vi "CRYView Queue.vi"() -> ()   [LabVIEW 2013]
uses:
  CRYView Global.vi
  SubVI/CRYMain Sub Window Global.vi
panel:
  in  "bVIRefRemove":bool=TRUE
  in  "ResultInCurLibrary":T1={"bResult"=TRUE, "SData_Out"="", "pVIRef_Out"=refnum, "pRefList_Out"=[]}
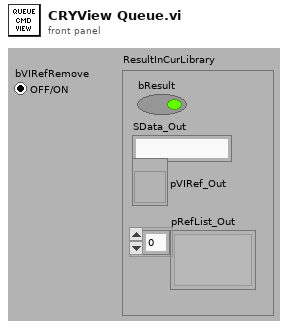
[diagram p1: front panel]
types:
  T1 = cluster{"bResult":bool, "SData_Out":string, "pVIRef_Out":refnum<vi>, "pRefList_Out":variant[]}
  T2 = cluster{"sCmdType":string, "nIDView":i32, "sAction":string, "sData":string, "sOption":string, "nData":i32, "nOption":i32, "pVIRef":refnum<vi>, "pSPRef":refnum<vi>, "bWaitRef":refnum<vi>, "Result":variant}[]
  T3 = cluster{"sCmdType":string, "nIDView":i32, "sAction":string, "sData":string, "sOption":string, "nData":i32, "nOption":i32, "pVIRef":refnum<vi>, "pSPRef":refnum<vi>, "bWaitRef":refnum<vi>, "Result":variant}
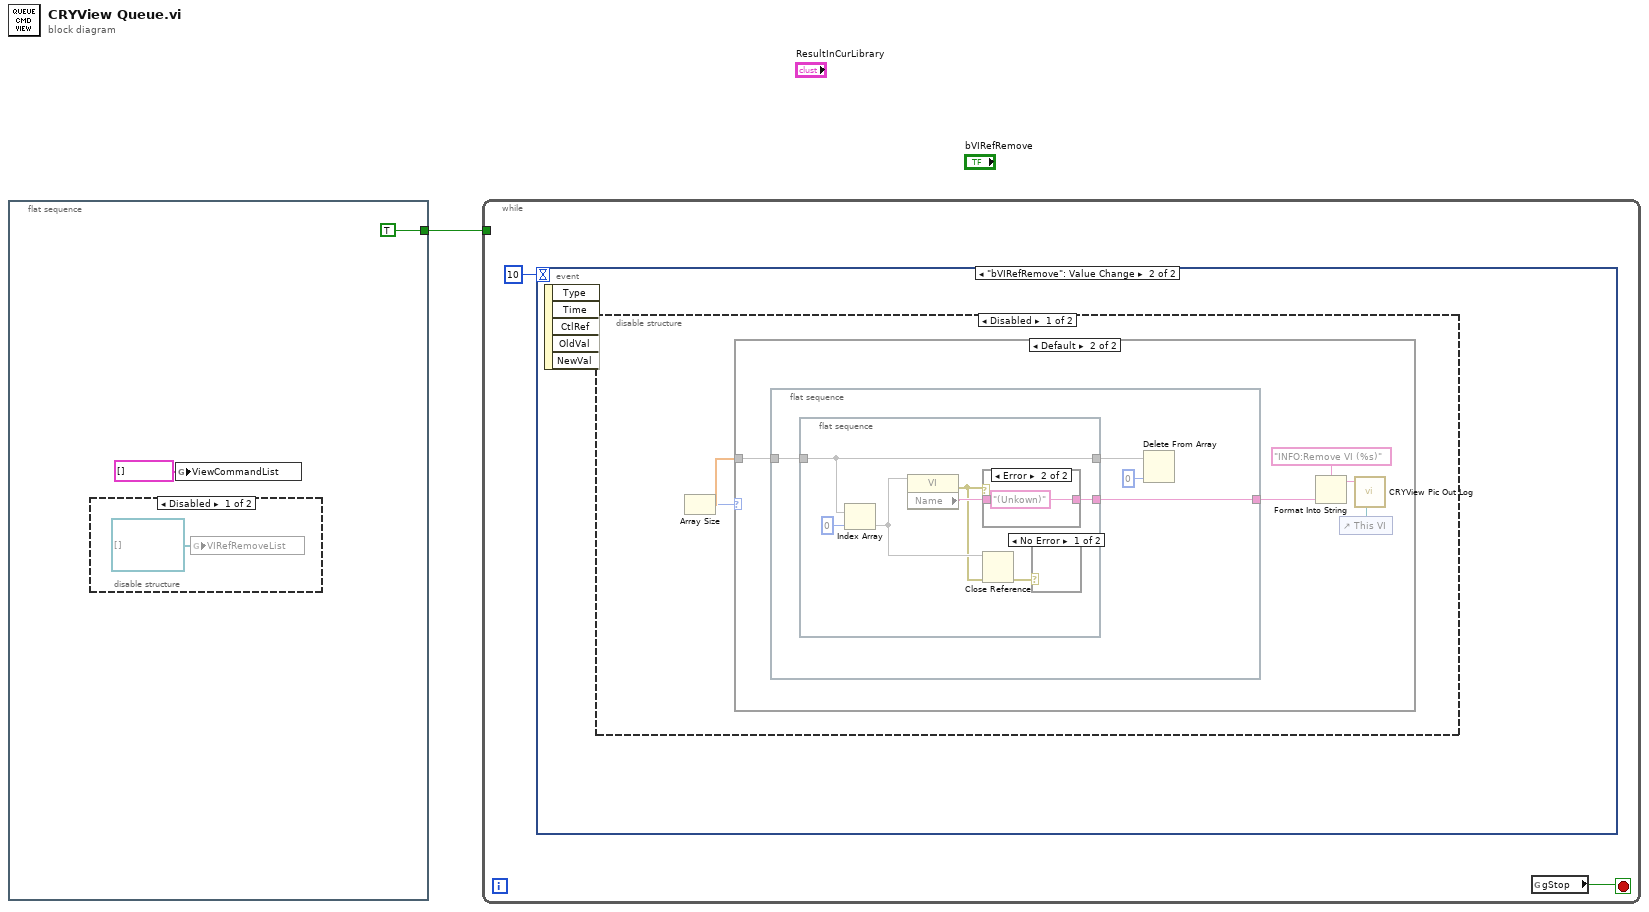
[diagram p0: block diagram]
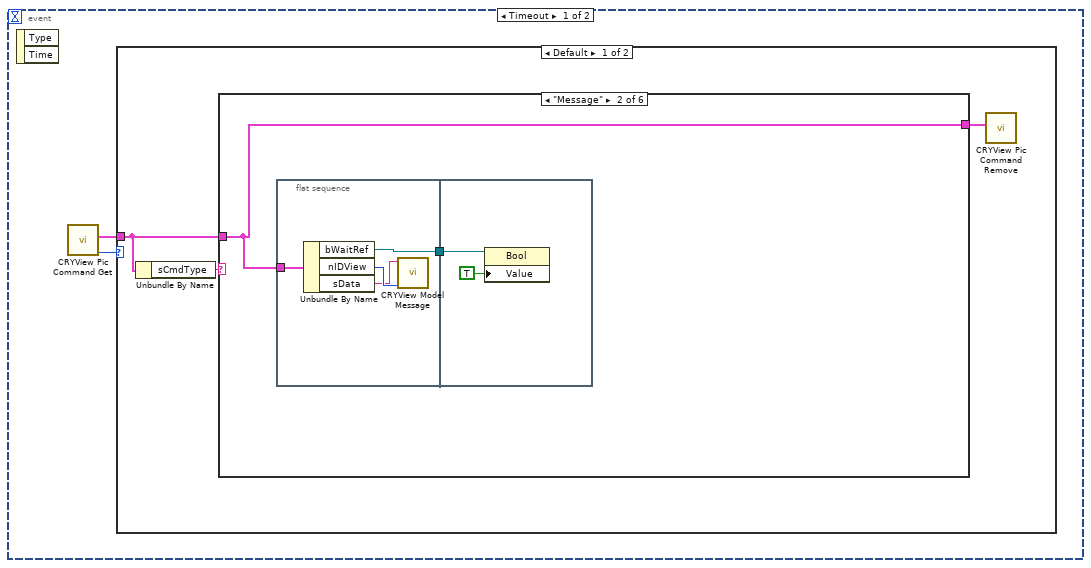
[diagram p3: hidden frame]
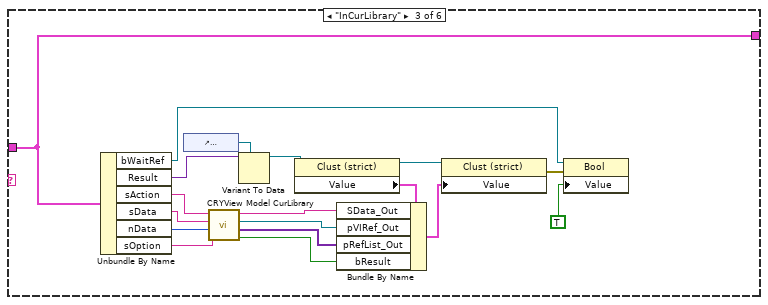
[diagram p5: hidden frame]
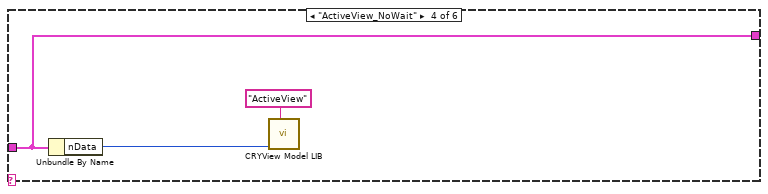
[diagram p6: hidden frame]
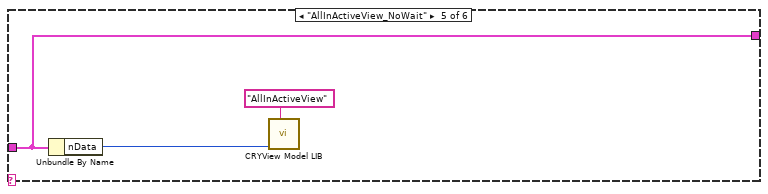
[diagram p7: hidden frame]
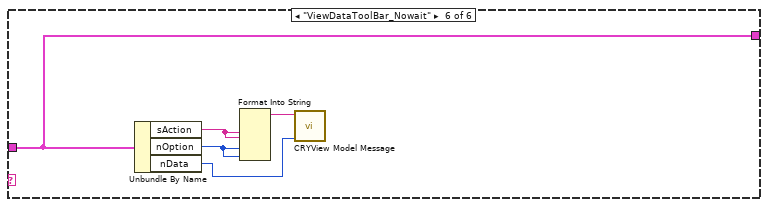
[diagram p8: hidden frame]
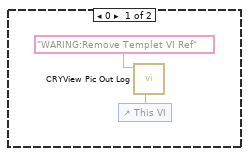
[diagram p10: hidden frame]
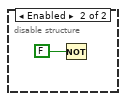
[diagram p13: hidden frame]
diagram:
  n1 = flat-sequence {
    tunnel: [TRUE] -> w1
    frame #0 {
      n2 = disable-structure shown="Disabled" {
        frame Disabled {
          n3 = global write "CRYView Global.vi" "VIRefRemoveList"(refnum<vi>[] [] ("VIRefRemoveList")) -> ()
        }
        frame Enabled {
        }
      }
      n4 = global write "CRYView Global.vi" "ViewCommandList"(T2 [] ("ViewCommandList")) -> ()
    }
  }
  n5 = while {
    tunnel: w1 -> [_]
    stop <- w5 stop-if-true
    n6 = event shown="[1] \"bVIRefRemove\": Value Change" {
      selector: _ -> [_ _]
      dyn-events: _ -> [_ _]
      timeout: 10 -> [_ _]
      event Timeout {
        n7 = event-data() -> ()  [unwired: 1 in, 2 out]
        n8 = call "CRYView Pic  Command Get.vi"() -> ("nData_Out"=w8:i32, "cCommand_Out"=w7:T3)  [unwired: 10 in]
        n9 = case shown="Default" w8 {
          tunnel: w7 -> [w10 _]
          frame Default {
            n10 = Unbundle By Name(w10) -> ("sCmdType"=w11:string)
            n11 = case shown="\"Message\"" w11 {
              tunnel: w10 -> [w12 w13 w21 w39 w42 w45]
              tunnel: [w12 w13 w21 w39 w42 w45] -> w9
              frame Default {
              }
              frame "Message" {
                n12 = flat-sequence {
                  tunnel: w13 -> [w16]
                  tunnel: [w15] -> w14
                  tunnel: w14 -> [w19]
                  frame #0 {
                    n13 = Unbundle By Name(w16) -> ("bWaitRef"=w15:refnum<vi>, "nIDView"=w18:i32, "sData"=w17:string)
                    n14 = call "CRYView Model Message.vi"("nData"=w18, "sMsgData"=w17) -> ()  [unwired: 7 in, 3 out]
                  }
                  frame #1 {
                    n15 = property class="Bool"(reference=w19, "Value"=TRUE) -> ()  [unwired: 1 in, 2 out]
                  }
                }
              }
              frame "InCurLibrary" {
                n16 = Unbundle By Name(w21) -> ("bWaitRef"=w22:refnum<vi>, "Result"=w34:variant, "sAction"=w38:string, "sData"=w37:string, "nData"=w36:i32, "sOption"=w35:string)
                n17 = control-ref of="ResultInCurLibrary"() -> (w33:refnum<vi>)
                n18 = call "CRYView Model CurLibrary.vi"("sOption"=w35, "nData"=w36, "sData"=w37, "sAction"=w38) -> ("bResult"=w27:bool, "pRefList_Out"=w28:variant[], "pVIRef_Out"=w29:refnum<vi>, "SData_Out"=w30:string)  [unwired: 4 in]
                n19 = Variant To Data(type=w33, Variant=w34) -> (data=w32:refnum<vi>)  [unwired: 1 in, 1 out]
                n20 = property class="Clust (strict)"(reference=w32) -> (reference out=w26:refnum<vi>, "Value"=w31:T1)  [unwired: 1 in, 1 out]
                n21 = Bundle By Name(cluster=w31, "SData_Out"=w30, "pVIRef_Out"=w29, "pRefList_Out"=w28, "bResult"=w27) -> (w25:T1)
                n22 = property class="Clust (strict)"(reference=w26, "Value"=w25) -> (error out=w23:errorcluster)  [unwired: 1 in, 1 out]
                n23 = property class="Bool"(reference=w22, error in=w23, "Value"=TRUE) -> ()  [unwired: 2 out]
              }
              frame "ActiveView_NoWait" {
                n24 = Unbundle By Name(w39) -> ("nData"=w40:i32)
                n25 = call "CRYView Model LIB.vi"("sAction"="ActiveView", "nData"=w40) -> ()  [unwired: 7 in, 3 out]
              }
              frame "AllInActiveView_NoWait" {
                n26 = Unbundle By Name(w42) -> ("nData"=w43:i32)
                n27 = call "CRYView Model LIB.vi"("sAction"="AllInActiveView", "nData"=w43) -> ()  [unwired: 7 in, 3 out]
              }
              frame "ViewDataToolBar_Nowait" {
                n28 = Unbundle By Name(w45) -> ("sAction"=w48:string, "nOption"=w47:i32, "nData"=w46:i32)
                n29 = Format Into String(w48, w48, w47, w47) -> (resulting string=w49:string)  [unwired: 3 in, 1 out]
                n30 = call "CRYView Model Message.vi"("nData"=w46, "sMsgData"=w49) -> ()  [unwired: 7 in, 3 out]
              }
            }
            n31 = call "CRYView Pic Command Remove.vi"("cCommand"=w9) -> ()  [unwired: 11 in]
          }
          frame 0 {
          }
        }
      }
      event "bVIRefRemove": Value Change {
        n32 = event-data() -> ()  [unwired: 1 in, 5 out]
        n33 = disable-structure shown="Disabled" {
          frame Disabled {
            n34 = Array Size() -> (array=w51:dbl[], size(s)=w50:i32)
            n35 = case shown="Default" w50 {
              tunnel: w51 -> [_ w58]
              frame 0 {
                n36 = control-ref of="This VI"() -> (w53:refnum<vi>)
                n37 = call "CRYView Pic Out Log.vi"("vi reference"=w53, "sData"="WARING:Remove Templet VI Ref") -> ()  [unwired: 10 in]
              }
              frame Default {
                n38 = flat-sequence {
                  tunnel: w58 -> [w60]
                  tunnel: [w59] -> w54
                  frame #0 {
                    n39 = flat-sequence {
                      tunnel: w60 -> [w68]
                      tunnel: [w68] -> w61
                      tunnel: [w64] -> w59
                      frame #0 {
                        n40 = Index Array(array=w68, index=0) -> (element=w66)
                        n41 = property class="VI"(reference=w66) -> (error out=w63:errorcluster, "Name"=w65:string)  [unwired: 1 in, 1 out]
                        n42 = case shown="Error" w63 {
                          tunnel: w65 -> [w70 _]
                          tunnel: [w70 "(Unkown)" ("Name")] -> w64
                          frame No Error {
                          }
                          frame Error {
                          }
                        }
                        n43 = Close Reference(reference=w66, error in (no error)=w63) -> (error out=w67:errorcluster)
                        n44 = case shown="No Error" w67 {
                          frame No Error {
                          }
                          frame Error {
                          }
                        }
                      }
                    }
                    n45 = Delete From Array(array=w61, index=0) -> ()  [unwired: 1 in, 2 out]
                  }
                }
                n46 = Format Into String(format string="INFO:Remove VI (%s)" ("sData"), w54) -> (resulting string=w56:string)  [unwired: 2 in, 1 out]
                n47 = control-ref of="This VI"() -> (w57:refnum<vi>)
                n48 = call "CRYView Pic Out Log.vi"("vi reference"=w57, "sData"=w56) -> ()  [unwired: 10 in]
              }
            }
          }
          frame Enabled {
            n49 = Not(x=FALSE) -> ()  [unwired: 1 out]
          }
        }
      }
    }
    n50 = global read "CRYMain Sub Window Global.vi" "gStop"() -> (w5:bool)
  }
